vi "Publish Trace.vi"(8 "error in (no error)":errorcluster, 10 "Trace In":refnum<class "Trace.lvclass">, 11 "System Actor in":refnum<class "System Actor.lvclass">) -> (0 "error out":errorcluster, 3 "System Actor out":refnum<class "System Actor.lvclass">)   [LabVIEW 2014, in "Robot Actor Framework.lvlib" / "System Actor.lvlib" / "System Actor.lvclass"]
uses:
  System Actor.lvclass
  Trace/Trace Class/Trace.lvclass
  System Actor.lvclass/System Actor.ctl
  <vilib>/ActorFramework/Message Enqueuer/Message Priority.ctl
  Trace/Trace Controller Messages/Publish Trace Msg/Publish Trace Msg.lvclass/Publish Trace Msg.ctl
  <vilib>/ActorFramework/Message Enqueuer/Message Enqueuer.lvclass/Message Enqueuer.ctl
  <vilib>/ActorFramework/Message Enqueuer/Enqueue.vi
  <vilib>/ActorFramework/Message Priority Queue/Priority Enqueue.vi
  Trace/Trace Controller Messages/Publish Trace Msg/Publish Trace Msg.lvclass
  <vilib>/ActorFramework/Message Enqueuer/Message Enqueuer.lvclass
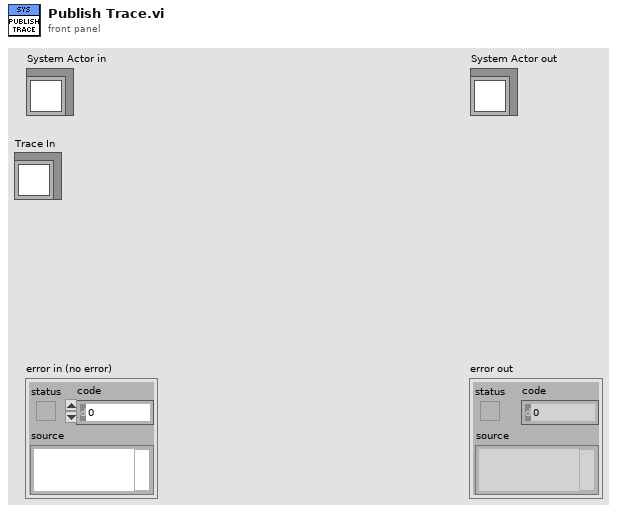
[diagram p1: front panel]
types:
  T1 = typedef "Robot Actor Framework.lvlib/Trace.lvlib/Trace.lvclass/Trace Levels.ctl" = enum16{"Critical", "Error", "Warning", "Informational", "Debug"}
  T2 = enum16{"Critical", "Error", "Warning", "Informational", "Debug"}
  T3 = typedef "Actor Framework.lvlib/Message Enqueuer.lvclass/Message Priority.ctl" = enum16{"Low", "Normal", "High"}
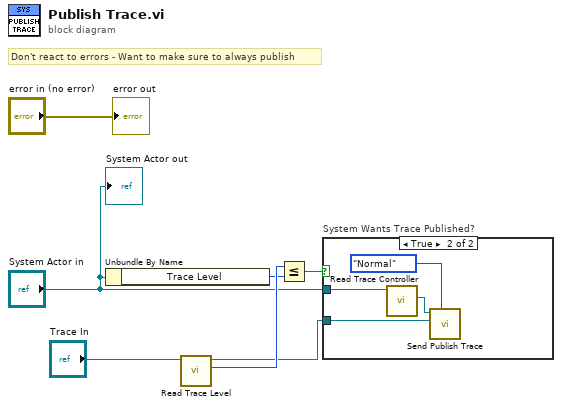
[diagram p0: block diagram]
diagram:
  # "Don't react to errors - Want to make sure to always publish"
  n1 = Unbundle By Name("System Actor in") -> ("Trace Level"=w1:T1)
  n2 = call-dynamic "Read Trace Level.vi"("Trace in"="Trace In") -> ("Trace Level"=w5:T2, "Trace out"=w3:refnum<class "Trace.lvclass">)  [unwired: 8 in, 1 out]
  n3 = Less Or Equal?(x=w5, y=w1) -> (x <= y?=w4:bool)
  n4 = case "System Wants Trace Published?" shown="True" w4 {
    tunnel: "System Actor in" -> [_ w11]
    tunnel: w3 -> [_ w8]
    frame False {
    }
    frame True {
      n5 = call-dynamic "Read Trace Controller.vi"("System Actor in"=w11) -> ("Trace Controller"=w10:refnum<class "Message Enqueuer.lvclass">)  [unwired: 8 in, 2 out]
      n6 = call "Send Publish Trace.vi"("Message Priority (Normal)"=Message_Priority."Normal", "Trace"=w8, "Message Enqueuer"=w10) -> ()  [unwired: 7 in, 2 out]
    }
  }
  "error out" <- "error in (no error)"
  "System Actor out" <- "System Actor in"
